vi "FRA example (A).vi"() -> ()   [LabVIEW 2011]
uses:
  C:/Program Files/Metrohm Autolab/Autolab SDK 1.10/EcoChemie.Autolab.Sdk.dll
  EcoChemie.Autolab.Sdk.dll
panel:
  out "-Z''":dbl[](array[numeric])
  out "-Phase":dbl[](array[numeric])
  out "Frequency":dbl[](array[numeric])
  out "Z'":dbl[](array[numeric])
  out "Z":dbl[](array[numeric])
  in  "load":bool
  out "Contains":bool
  out "Bode phase":cluster{"Y":dbl[], "Y":dbl[]}[](graph)
  out "E & I":cluster{"Y":dbl[], "Y":dbl[]}[](graph)
  in  "Save":bool
  in  "Path":string
  in  "Hardware Setup File":path
  in  "Embedded Exe File":path
  in  "Path":path=path "Standard Nova Procedures/FRA impedance potentiostatic.nox"
  out "error out":errorcluster
  out "Nyquist":cluster{"Y":dbl[], "Y":dbl[]}[](graph)
  out "Bode Z":cluster{"Y":dbl[], "Y":dbl[]}[](graph)
  out "Ismeasuring":bool
  in  "abort":bool
  in  "stop":bool
  in  "Start Measure":bool
  out "IsConnected":bool
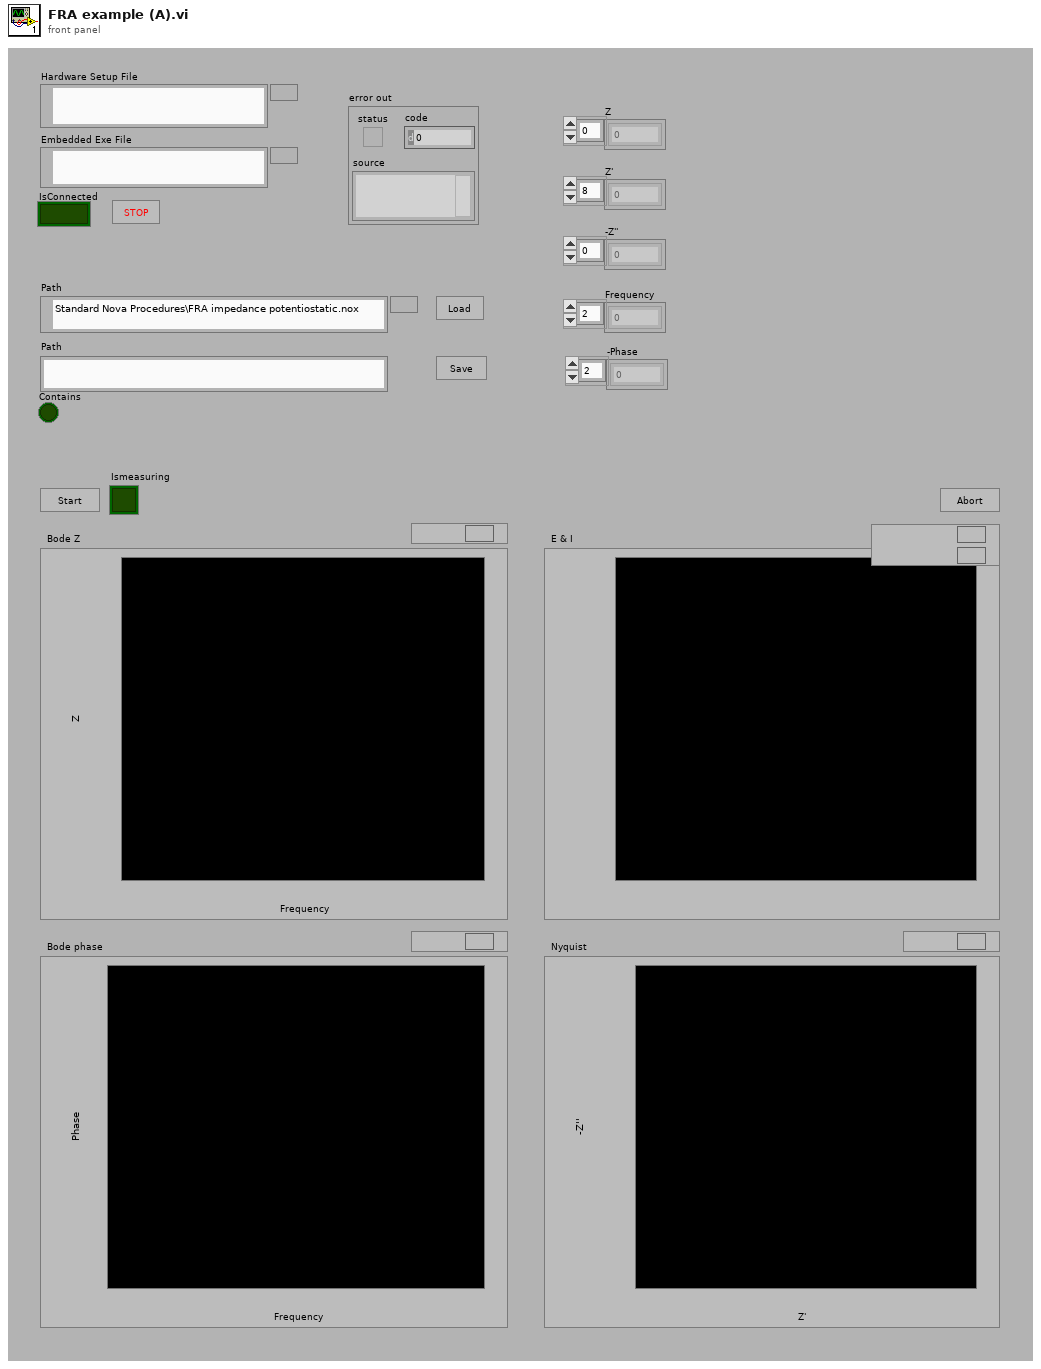
[diagram p1: front panel]
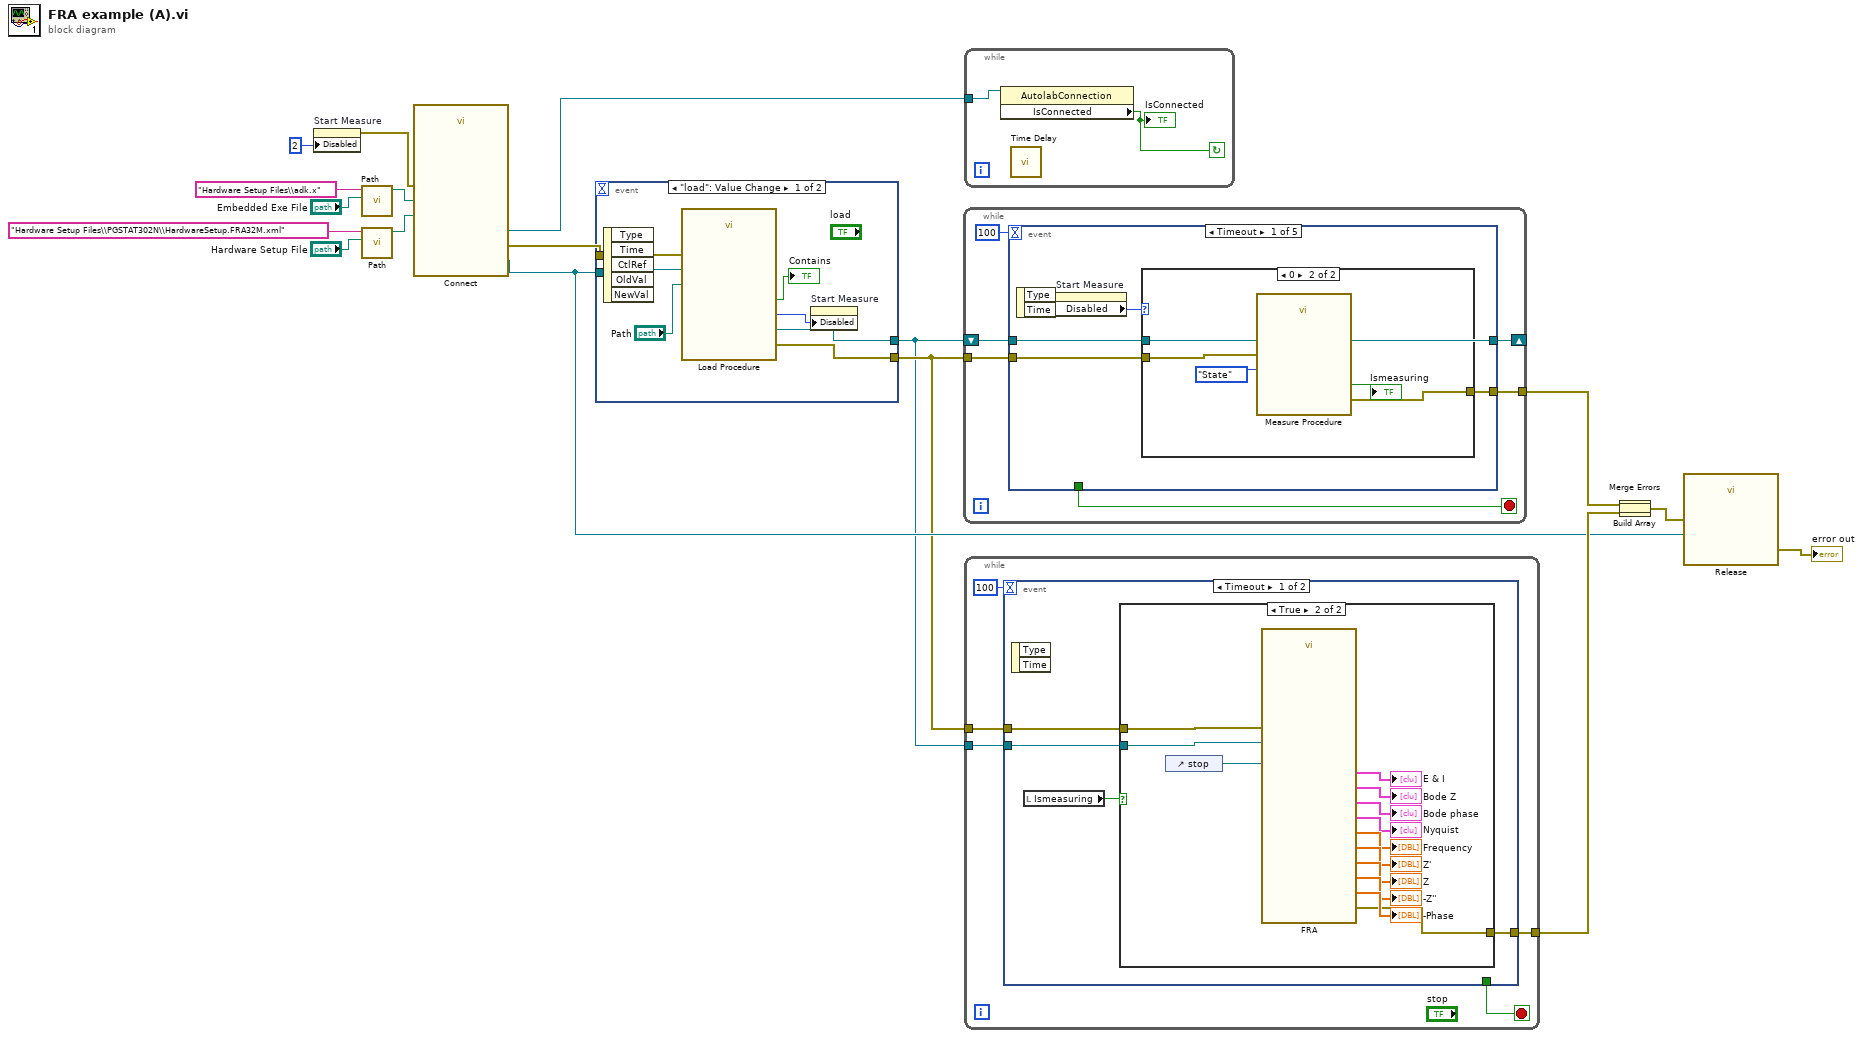
[diagram p0: block diagram]
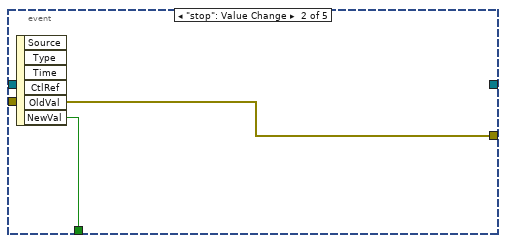
[diagram p3: hidden frame]
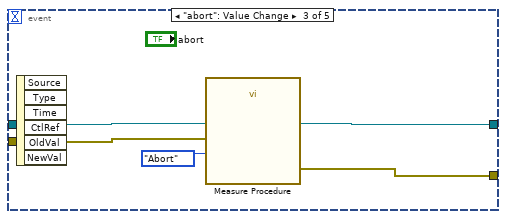
[diagram p4: hidden frame]
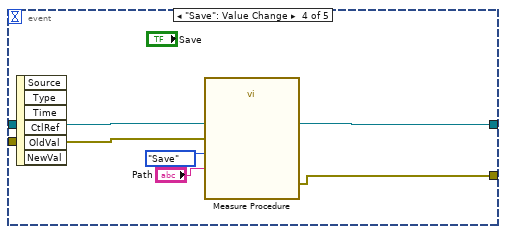
[diagram p5: hidden frame]
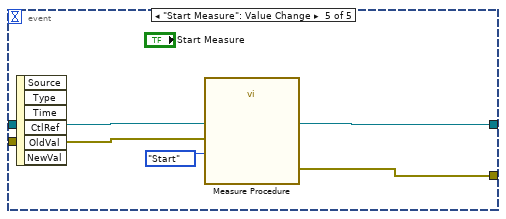
[diagram p6: hidden frame]
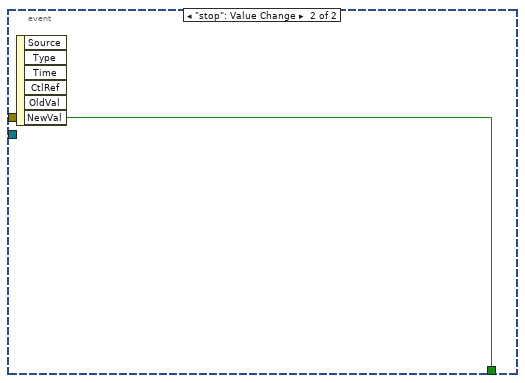
[diagram p8: hidden frame]
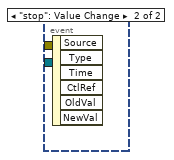
[diagram p9: hidden frame]
diagram:
  n1 = property on="Start Measure" class="Bool"("Disabled"=u8 2) -> (error out=w5:errorcluster)  [unwired: 2 in, 1 out]
  n2 = call "Path.vi"("File"="Embedded Exe File", "name or relative path"="Hardware Setup Files\\adk.x") -> ("appended path"=w9:path)  [unwired: 9 in]
  n3 = call "Path.vi"("File"="Hardware Setup File", "name or relative path"="Hardware Setup Files\\PGSTAT302N\\HardwareSetup.FRA32M.xml") -> ("appended path"=w8:path)  [unwired: 9 in]
  n4 = call "Connect.vi"("Embedded Exe File"=w9, "Hardware Setup File"=w8, "error in (no error)"=w5) -> ("AutolabConnection"=w2:refnum<k24>, "instrument"=w13:refnum<k24>, "error out"=w18:errorcluster)  [unwired: 5 in, 5 out]
  n5 = event shown="[0] \"load\": Value Change" {
    selector: _ -> [_ _]
    dyn-events: _ -> [_ _]
    timeout: _ -> [_ _]
    tunnel: w18 -> [w25 _]
    tunnel: w13 -> [w24 _]
    tunnel: [w21 _] -> w3
    tunnel: [w20 _] -> w12
    event "load": Value Change {
      n6 = event-data() -> ()  [unwired: 1 in, 5 out]
      n7 = call "Load Procedure.vi"("error in (no error)"=w25, "Procedure"="Path", "Instrument"=w24) -> ("error out"=w20:errorcluster, "Contains"=→"Contains":bool, "Numeric"=w19:i32, "LoadProcedure"=w21:refnum<k24>)  [unwired: 5 in]
      n8 = property on="Start Measure" class="Bool"("Disabled"=w19) -> ()  [unwired: 2 in, 2 out]
    }
    event "stop": Value Change {
      n9 = event-data() -> ()  [unwired: 1 in, 6 out]
    }
  }
  n10 = while {
    shift-right: [w29] -> _
    shift-left: w3 -> [w30]
    tunnel: w12 -> [w28]
    tunnel: [w26] -> w15
    stop <- w31 stop-if-true
    n11 = event shown="[0] Timeout" {
      selector: _ -> [_ _ _ _ _]
      dyn-events: _ -> [_ _ _ _ _]
      timeout: 100 -> [_ _ _ _ _]
      tunnel: [_ w43 _ _ _] -> w31
      tunnel: w30 -> [w32 _ w44 w50 w54]
      tunnel: [w32 _ w44 w50 w54] -> w29
      tunnel: w28 -> [w34 w42 w47 w49 w55]
      tunnel: [w33 w42 w45 w48 w53] -> w26
      event Timeout {
        n12 = event-data() -> ()  [unwired: 1 in, 2 out]
        n13 = property on="Start Measure" class="Bool"() -> ("Disabled"=w35:u8)  [unwired: 2 in, 2 out]
        n14 = case shown="0" w35 {
          tunnel: w32 -> [_ w39]
          tunnel: w34 -> [w36 w38]
          tunnel: [w36 w37] -> w33
          frame 2, Default {
          }
          frame 0 {
            n15 = call "Measure Procedure.vi"("error in"=w38, "Request for procedure"=enum16{"State", "Save", "Abort", "Start"}."State", "LoadProcedure"=w39) -> ("error out"=w37:errorcluster, "IsMeasuring"=→"Ismeasuring":bool)  [unwired: 7 in]
          }
        }
      }
      event "stop": Value Change {
        n16 = event-data() -> ("NewVal"=w43:bool)  [unwired: 1 in, 5 out]
      }
      event "abort": Value Change {
        n17 = event-data() -> ()  [unwired: 1 in, 6 out]
        n18 = call "Measure Procedure.vi"("error in"=w47, "Request for procedure"=enum16{"State", "Save", "Abort", "Start"}."Abort", "LoadProcedure"=w44) -> ("error out"=w45:errorcluster)  [unwired: 7 in, 1 out]
      }
      event "Save": Value Change {
        n19 = event-data() -> ()  [unwired: 1 in, 6 out]
        n20 = call "Measure Procedure.vi"("error in"=w49, "fileName"="Path", "Request for procedure"=enum16{"State", "Save", "Abort", "Start"}."Save", "LoadProcedure"=w50) -> ("error out"=w48:errorcluster)  [unwired: 6 in, 1 out]
      }
      event "Start Measure": Value Change {
        n21 = event-data() -> ()  [unwired: 1 in, 6 out]
        n22 = call "Measure Procedure.vi"("error in"=w55, "Request for procedure"=enum16{"State", "Save", "Abort", "Start"}."Start", "LoadProcedure"=w54) -> ("error out"=w53:errorcluster)  [unwired: 7 in, 1 out]
      }
    }
  }
  n23 = while {
    tunnel: w2 -> [w57]
    stop <- w58 continue-if-true
    n24 = property class="AutolabConnection"(reference=w57) -> ("IsConnected"=w58:bool)  [unwired: 1 in, 2 out]
    "IsConnected" <- w58
    n25 = call "Time Delay"() -> ()  [unwired: 11 in, 1 out]
  }
  n26 = while {
    tunnel: [w62] -> w14
    tunnel: w12 -> [w61]
    tunnel: w3 -> [w59]
    stop <- w63 stop-if-true
    n27 = event shown="[0] Timeout" {
      selector: _ -> [_ _]
      dyn-events: _ -> [_ _]
      timeout: 100 -> [_ _]
      tunnel: [_ w82] -> w63
      tunnel: [w67 _] -> w62
      tunnel: w61 -> [w66 _]
      tunnel: w59 -> [w65 _]
      event Timeout {
        n28 = event-data() -> ()  [unwired: 1 in, 2 out]
        n29 = local read "Ismeasuring"() -> (w64:bool)
        n30 = case shown="True" w64 {
          tunnel: [w68 w71] -> w67
          tunnel: w66 -> [w68 w70]
          tunnel: w65 -> [_ w69]
          frame False {
          }
          frame True {
            n31 = control-ref of="stop"() -> (w72:refnum<vi>)
            n32 = call "FRA.vi"("LoadProcedure"=w69, "stop"=w72, "error in"=w70) -> ("Bode phase"=→"Bode phase":cluster{"Y":dbl[], "Y":dbl[]}[], "Bode Z"=→"Bode Z":cluster{"Y":dbl[], "Y":dbl[]}[], "Nyquist"=→"Nyquist":cluster{"Y":dbl[], "Y":dbl[]}[], "E & I"=→"E & I":cluster{"Y":dbl[], "Y":dbl[]}[], "-Phase"=→"-Phase":dbl[], "Frequency"=→"Frequency":dbl[], "-Z''"=→"-Z''":dbl[], "Z"=→"Z":dbl[], "Z'"=→"Z'":dbl[], "error out"=w71:errorcluster)  [unwired: 15 in]
          }
        }
      }
      event "stop": Value Change {
        n33 = event-data() -> ("NewVal"=w82:bool)  [unwired: 1 in, 5 out]
      }
    }
  }
  n34 = Build Array(w15, w14) -> (w1:errorcluster[])
  n35 = Merge Errors(w1) -> (w17:errorcluster)
  n36 = call "Release.vi"("error in (no error)"=w17, "Instrument"=w13) -> ("error out"=→"error out":errorcluster)  [unwired: 9 in]
